vi "MFLI_File_write.vi"(6 "Type (text)":enum16{"bin", "text"}(ring)=enum."text", 7 "String":string, 8 "Error In":errorcluster, 9 "access (0:read/write)":enum16{"read/write", "read-only", "write-only"}(ring), 10 "operation (0:open)":T1(ring), 11 "selected path":path) -> (0 "Error Out":errorcluster, 3 "selected path out":path)   [LabVIEW 2018]
uses:
  <vilib>/addons/Tools/Unicode/UTF8 Tools.lvlib
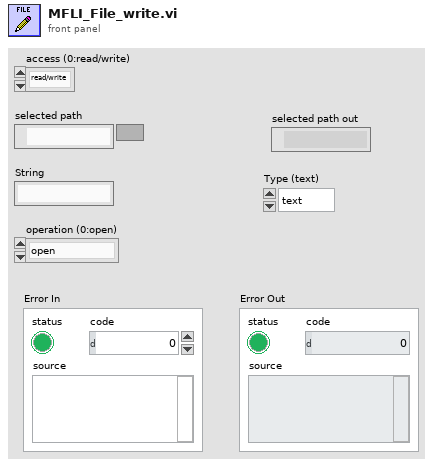
[diagram p1: front panel]
types:
  T1 = enum16{"open", "replace", "create", "open or create", "replace or create", "replace or create with confirmation"}
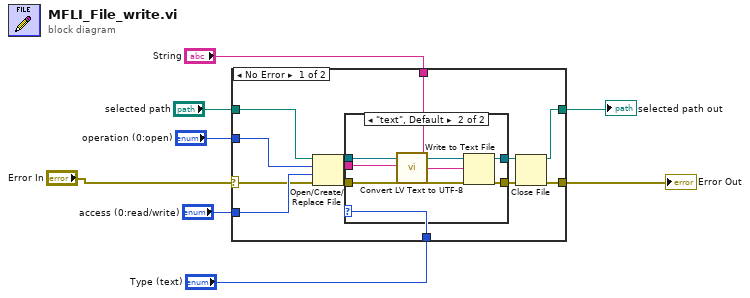
[diagram p0: block diagram]
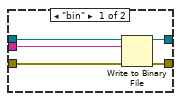
[diagram p2: hidden frame]
diagram:
  n1 = case shown="No Error" "Error In" {
    selector: "Error In" -> [w13 w33]
    tunnel: "operation (0:open)" -> [w20 _]
    tunnel: "access (0:read/write)" -> [w19 _]
    tunnel: [w10 w33] -> w1
    tunnel: "String" -> [w16 _]
    tunnel: "Type (text)" -> [w15 _]
    tunnel: "selected path" -> [w14 w32]
    tunnel: [w9 w32] -> w3
    frame No Error {
      n2 = Open/Create/Replace File(file path (use dialog)=w14, error in=w13, operation (0:open)=w20, access (0:read/write)=w19) -> (refnum out=w17:refnum<file>, error out=w18:errorcluster)  [unwired: 2 in, 1 out]
      n3 = case shown="\"text\", Default" w15 {
        tunnel: [w22 w31] -> w11
        tunnel: [w24 w30] -> w12
        tunnel: w18 -> [w25 w29]
        tunnel: w17 -> [w23 w28]
        tunnel: w16 -> [w21 w27]
        frame "bin" {
          n4 = Write to Binary File(file (use dialog)=w23, data=w21, error in=w25) -> (refnum out=w22:refnum<file>, error out=w24:errorcluster)  [unwired: 3 in, 1 out]
        }
        frame "text", Default {
          n5 = call <vilib>:"Convert LV Text to UTF-8.vi"("LV Text"=w27) -> ("UTF-8 Text"=w26:string)  [unwired: 13 in, 1 out]
          n6 = Write to Text File(file (use dialog)=w28, text=w26, error in=w29) -> (refnum out=w31:refnum<file>, error out=w30:errorcluster)  [unwired: 1 in, 1 out]
        }
      }
      n7 = Close File(refnum=w11, error in=w12) -> (path=w9:path, error out=w10:errorcluster)
    }
    frame Error {
    }
  }
  "selected path out" <- w3
  "Error Out" <- w1
